vi "Initialize Data Ref.vi"(8 "error in (no error)":errorcluster, 10 "Data Ref":T1, 11 "VeriStand DSF in":refnum<class "VeriStand DSF.lvclass">) -> (0 "error out":errorcluster, 3 "VeriStand DSF out":refnum<class "VeriStand DSF.lvclass">)   [LabVIEW 2017, in "DSF Engine.lvlib" / "VeriStand DSF.lvclass"]
uses:
  VeriStand DSF.lvclass
  <vilib>/NI Veristand/Custom Device API/Data Table Ref.ctl
  DSF Core.lvlibp/Classes/Framework/Framework.lvclass
  C:/Git/DSF/VeriStand/Data Sharing Custom Device/Source/DSF Core.lvlibp/Classes/Framework/Framework.lvclass
  <vilib>/NI Veristand/Custom Device API/Custom Device API.lvlib
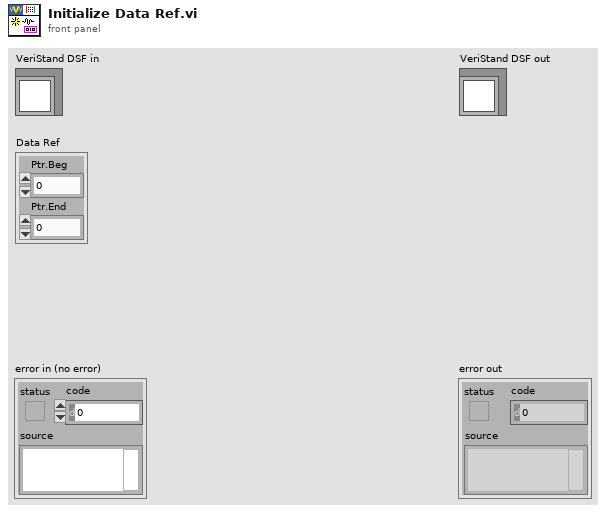
[diagram p1: front panel]
types:
  T1 = typedef "Custom Device API.lvlib/Data Table Ref.ctl" = cluster{"Ptr.Beg":u64, "Ptr.End":u64}
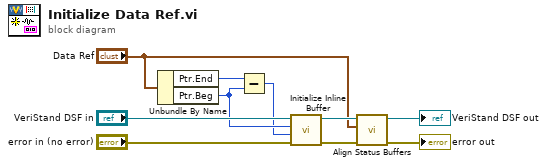
[diagram p0: block diagram]
diagram:
  n1 = Unbundle By Name("Data Ref") -> ("Ptr.End"=w8:u64, "Ptr.Beg"=w7:u64)
  n2 = Subtract(x=w8, y=w7) -> (x-y=w6:u64)
  n3 = call "Initialize Inline Buffer.vi"("error in (no error)"="error in (no error)", "size"=w6, "address"=w7, "Framework in"="VeriStand DSF in") -> ("error out"=w5:errorcluster, "Framework out"=w4:refnum<class "VeriStand DSF.lvclass">)  [unwired: 6 in]
  n4 = call "Align Status Buffers.vi"("error in (no error)"=w5, "Data Ref"="Data Ref", "VeriStand DSF in"=w4) -> ("error out"=→"error out":errorcluster, "VeriStand DSF out"=→"VeriStand DSF out":refnum<class "VeriStand DSF.lvclass">)  [unwired: 7 in]
